vi "moveSlitMM.vi"(6 "Delay between send and receive [ms]":i32=100, 8 "error in (no error)":errorcluster, 9 "position":dbl format="%#_13g", 10 "locationId":i32, 11 "Monochromator in":refnum<class "Monochromator.lvclass">) -> (0 "error out":errorcluster, 1 "ID":i32, 2 "results-JSON string":string, 3 "Monochromator out":refnum<class "Monochromator.lvclass">)   [LabVIEW 2020, in "horiba.lvlib" / "Monochromator.lvclass"]
doc: "Moves the specified slit to the position in millimeters. The location id of each configured slit can be found under the ports section of the mono configuration. See mono_getConfig for additional information.\n\nlocationId Integer. Used to identify the slit location.\n1 = Front entrance (axial)\n2 = Side entrance (lateral)\n3 = Front exit (axial)\n4 = Side exit (lateral)\nFor example:\n\n\"ports\": [\n {\n \"locationId\": 1,\n \"slitType\": 1\n },\n {\n \"locationId\": 2,\n \"slitType\": 1\n },\n {\n \"locationId\": 4,\n \"slitType\": 1\n }\n]\nNote: The \"locationId\" parameter found in the mono configuration is 1-based. However, the mono_moveSlitMM command uses a 0-based \"locationId\".\n\nlocationId Integer. Slit location (zero-based)\nposition Float. Position in millimeters"
uses:
  Monochromator.lvclass
  Monochromator.lvclass/Monochromator.ctl
  f95066af-ee3f-403d-a38c-ce622af095b7.vi
  GenericDevice/GenericDevice.lvclass
  675900b5-fd1a-4005-b0fd-0124d8ccfa64.vi
  6615e9bd-2c56-4b02-b41e-62addde286d0.vi
panel:
  # "Connector Pane"
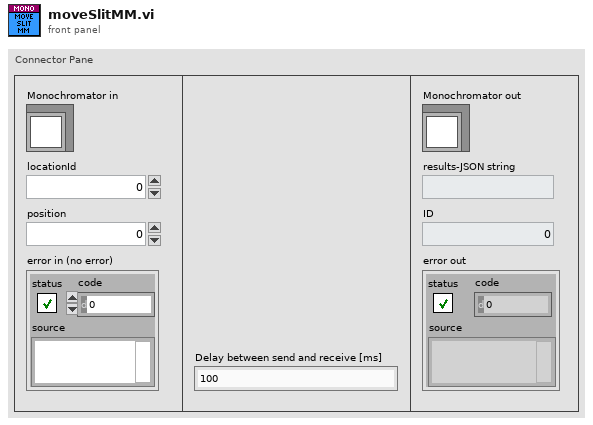
[diagram p1: front panel]
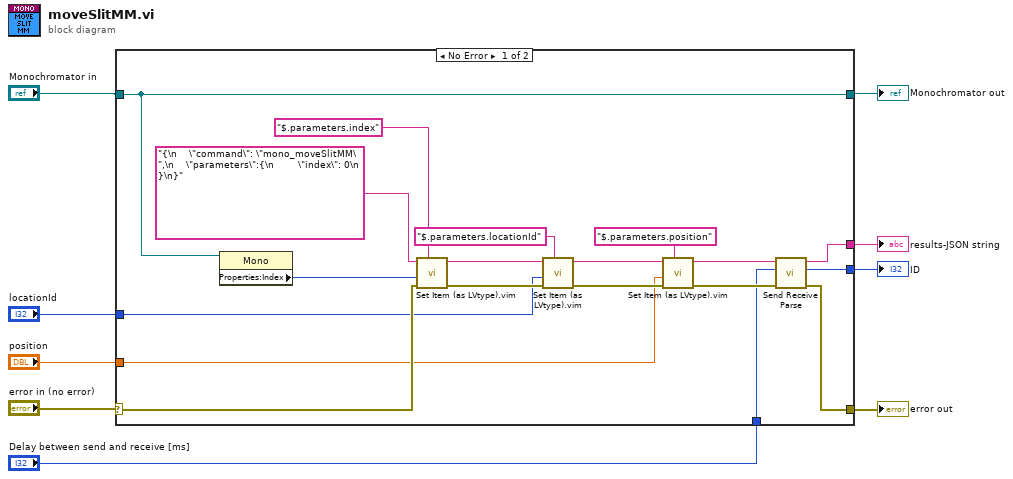
[diagram p0: block diagram]
diagram:
  n1 = case shown="No Error" "error in (no error)" {
    selector: "error in (no error)" -> [w24 w30]
    tunnel: [w21 w30] -> w6
    tunnel: [w26 w29] -> w8
    tunnel: "Monochromator in" -> [w26 w29]
    tunnel: [w23 _] -> w4
    tunnel: [w22 _] -> w5
    tunnel: "locationId" -> [w13 _]
    tunnel: "position" -> [w12 _]
    tunnel: "Delay between send and receive [ms]" -> [w11 _]
    frame No Error {
      n2 = property class="Mono"(reference=w26) -> ("Properties:Index"=w25:i32)  [unwired: 1 in, 2 out]
      n3 = call "Set Item (as LVtype).vim"("$Path or Item Name"="$.parameters.index", "error in (no error)"=w24, "Anything"=w25, "JSON"="{\n    \"command\": \"mono_moveSlitMM\",\n    \"parameters\":{\n        \"index\": 0\n    }\n}") -> ("error out"=w15:errorcluster, "<JSON>"=w17:string)  [unwired: 4 in, 1 out]
      n4 = call "Set Item (as LVtype).vim"("$Path or Item Name"="$.parameters.locationId", "error in (no error)"=w15, "Anything"=w13, "JSON"=w17) -> ("error out"=w14:errorcluster, "<JSON>"=w16:string)  [unwired: 4 in, 1 out]
      n5 = call "Set Item (as LVtype).vim"("$Path or Item Name"="$.parameters.position", "error in (no error)"=w14, "Anything"=w12, "JSON"=w16) -> ("error out"=w19:errorcluster, "<JSON>"=w10:string)  [unwired: 4 in, 1 out]
      n6 = call "Send Receive Parse.vi"("error in"=w19, "Delay between send and receive [ms]"=w11, "<JSON>"=w10) -> ("error out"=w21:errorcluster, "ID"=w22:i32, "results-JSON string"=w23:string)  [unwired: 6 in]
    }
    frame Error {
    }
  }
  "error out" <- w6
  "Monochromator out" <- w8
  "ID" <- w5
  "results-JSON string" <- w4
